vi "Agilent 3446X Series Acquire Triggered Multiple.vi"() -> ()   [LabVIEW 2015]
doc: "This example shows how to configure a measurement, set up triggering, trigger a measurement, and retrieve a measurement. It shows how to use the low-level Data VIs to retrieve data from the DMM."
uses:
  <instrlib>/Agilent 3446X Series/Agilent 3446X Series.lvlib
panel:
  in  "VISA resource name":refnum<visa-resource-name>
  in  "Timeout (10000 ms)":i32=10000 format="%#.6g"
  in  "Measurement Function (10: Voltage DC)":i32(ring)=10 items=["Continuity", "Current AC", "Current DC", "Diode", "Frequency", "Resistance 4-wire", "Period", "Resistance 2-wire", "Temperature", "Voltage AC", "Voltage DC", "Voltage DC Ratio"]
  in  "Trigger Count (1)":i32=1 format="%#.6g"
  in  "Sample Count (1)":i32=1 format="%#.6g"
  out "Waveform Chart":dbl[](graph)
  # "(c) 2013-2015 National Instruments.  ALL RIGHTS RESERVED."
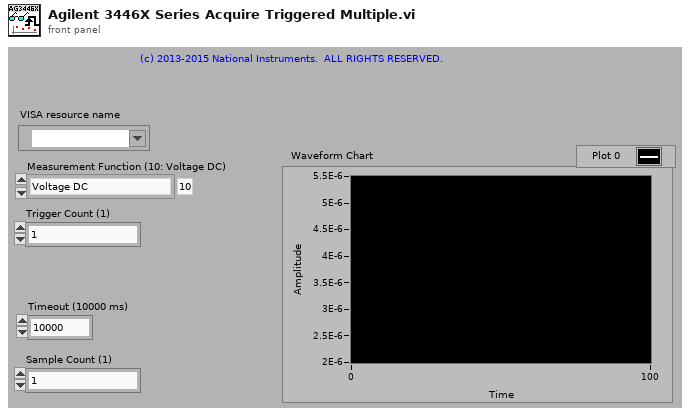
[diagram p1: front panel]
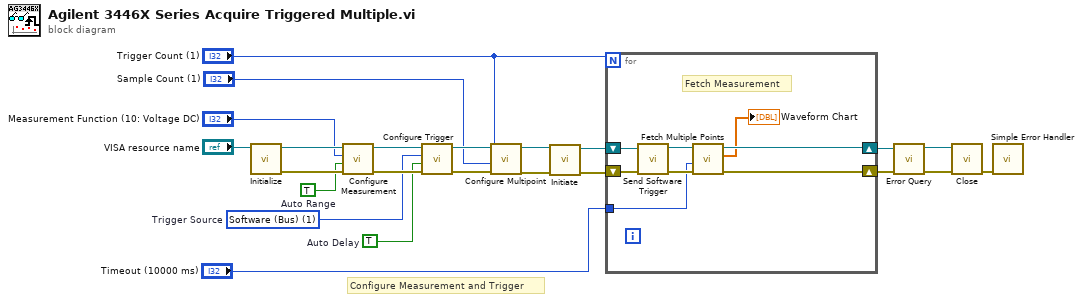
[diagram p0: block diagram]
diagram:
  w3 = 1 items=["Immediate", "Software (Bus)", "External"]  # Trigger Source
  w15 = TRUE  # Auto Range
  w16 = TRUE  # Auto Delay
  # "Configure Measurement and Trigger"
  n1 = call <instrlib>:"Initialize.vi"("VISA resource name"="VISA resource name") -> ("error out"=w22:errorcluster, "VISA resource name out"=w23:refnum<visa-resource-name>)  [unwired: 4 in, 5 out]
  n2 = call <instrlib>:"Configure Measurement.vi"("error in (no error)"=w22, "Auto Range (T: Enable)"=w15, "Measurement Function (10: Voltage DC)"="Measurement Function (10: Voltage DC)", "VISA resource name"=w23) -> ("error out"=w20:errorcluster, "VISA resource name out"=w21:refnum<visa-resource-name>)  [unwired: 2 in, 4 out]
  n3 = call <instrlib>:"Configure Trigger.vi"("error in (no error)"=w20, "Auto Delay (T:Enable)"=w16, "Trigger Source (0: Immediate)"=w3, "VISA resource name"=w21) -> ("error out"=w18:errorcluster, "VISA resource name out"=w19:refnum<visa-resource-name>)  [unwired: 2 in, 4 out]
  n4 = call <instrlib>:"Configure Multipoint.vi"("error in (no error)"=w18, "Sample Count (1)"="Sample Count (1)", "Trigger Count (1)"="Trigger Count (1)", "VISA resource name"=w19) -> ("error out"=w13:errorcluster, "VISA resource name out"=w14:refnum<visa-resource-name>)  [unwired: 3 in, 3 out]
  n5 = call <instrlib>:"Initiate.vi"("error in (no error)"=w13, "VISA resource name"=w14) -> ("error out"=w12:errorcluster, "VISA resource name out"=w11:refnum<visa-resource-name>)  [unwired: 8 out]
  n6 = for {
    N: "Trigger Count (1)" -> [_]
    shift-right: [w30] -> w8
    shift-left: w12 -> [w25]
    tunnel: "Timeout (10000 ms)" -> [w24]
    shift-right: [w31] -> w10
    shift-left: w11 -> [w26]
    # "Fetch Measurement"
    n7 = call <instrlib>:"Send Software Trigger.vi"("error in (no error)"=w25, "VISA resource name"=w26) -> ("error out"=w27:errorcluster, "VISA resource name out"=w28:refnum<visa-resource-name>)  [unwired: 8 out]
    n8 = call <instrlib>:"Fetch Multiple Points.vi"("error in (no error)"=w27, "Timeout (10000 ms)"=w24, "VISA resource name"=w28) -> ("error out"=w30:errorcluster, "Measurements"=→"Waveform Chart":dbl[], "VISA resource name out"=w31:refnum<visa-resource-name>)  [unwired: 1 in, 5 out]
  }
  n9 = call <instrlib>:"Error Query.vi"("error in (no error)"=w8, "VISA resource name"=w10) -> ("error out"=w7:errorcluster, "VISA resource name out"=w9:refnum<visa-resource-name>)  [unwired: 8 out]
  n10 = call <instrlib>:"Close.vi"("error in (no error)"=w7, "VISA resource name"=w9) -> ("error out"=w17:errorcluster)  [unwired: 9 out]
  n11 = call <vilib>:"Simple Error Handler.vi"("error in (no error)"=w17) -> ()  [unwired: 1 in, 8 out]
